vi "Determine Warning - efficient but not scalable.vi"(6 "High Wind Speed":dbl, 7 "Current Wind Speed":dbl, 8 "error in (no error)":errorcluster, 9 "Low Temp":dbl, 10 "High Temp":dbl, 11 "Current Temperature":dbl) -> (0 "error out":errorcluster, 1 "Warning?":bool, 2 "Warning Text":string)   [LabVIEW 2010]
doc: "This VI is one solution to an exercise in the LabVIEW Core II course. In this exercise, you take inherited code and improve it for readability and maintainability."
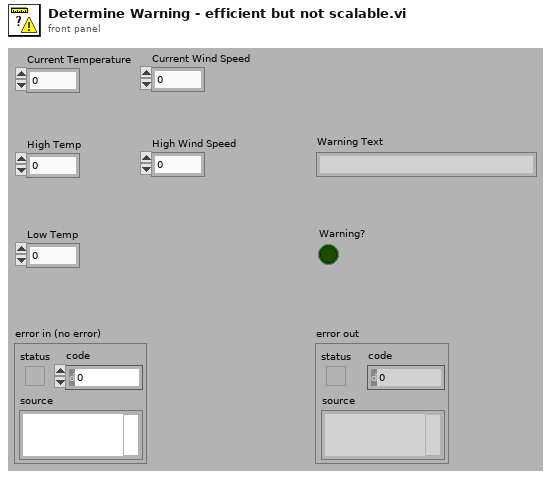
[diagram p1: front panel]
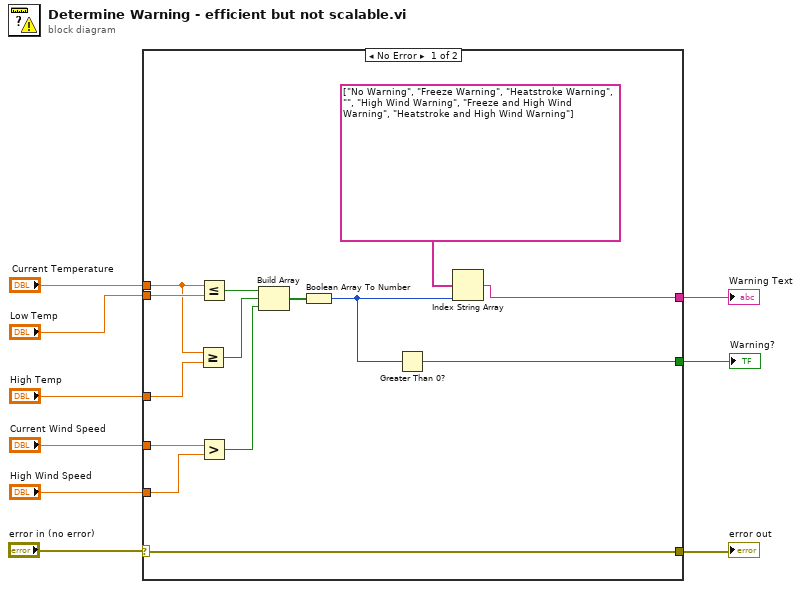
[diagram p0: block diagram]
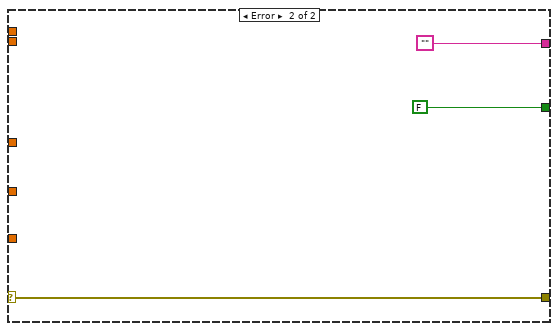
[diagram p2: hidden frame]
diagram:
  n1 = case shown="No Error" "error in (no error)" {
    selector: "error in (no error)" -> [w11 w26]
    tunnel: "High Temp" -> [w23 _]
    tunnel: "Low Temp" -> [w22 _]
    tunnel: "Current Wind Speed" -> [w21 _]
    tunnel: "High Wind Speed" -> [w20 _]
    tunnel: "Current Temperature" -> [w19 _]
    tunnel: [w13 ""] -> w4
    tunnel: [w12 FALSE] -> w3
    tunnel: [w11 w26] -> w1
    frame No Error {
      n2 = Greater Or Equal?(x=w19, y=w23) -> (x >= y?=w17:bool)
      n3 = Less Or Equal?(x=w19, y=w22) -> (x <= y?=w18:bool)
      n4 = Greater?(x=w21, y=w20) -> (0:w15:bool)
      n5 = Build Array(w18, w17, w15) -> (w16:bool[])
      n6 = Boolean Array To Number(Boolean array=w16) -> (number=w10:u32)
      n7 = Greater Than 0?(x=w10) -> (x > 0?=w12:bool)
      n8 = Index String Array(1:w10, 2:string[] ["No Warning", "Freeze Warning", "Heatstroke Warning", "", "High Wind Warning", "Freeze and High Wind Warning", "Heatstroke and High Wind Warning"]) -> (0:w13:string)  [unwired: 1 out]
    }
    frame Error {
    }
  }
  "error out" <- w1
  "Warning Text" <- w4
  "Warning?" <- w3
